vi "Test DataType Conversion.vi"() -> ()   [LabVIEW 2021]
uses:
  <vilib>/Utility/Data Type/Type Definitions/Data Type.ctl
  DataTypes_CIF_U.lvlib
  <vilib>/Utility/Data Type/NI_Data Type.lvlib
panel:
  out "Pass":bool
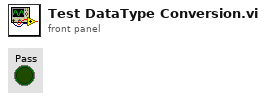
[diagram p1: front panel]
types:
  T1 = typedef "NI_Data Type.lvlib/Data Type.ctl" = enum8{"Invalid Type", "Void", "I8", "I16", "I32", "I64", "U8", "U16", "U32", "U64", "Single Float", "Double Float", "Extended Float", "Single Complex", "Double Complex", "Extended Complex", "Enum U8", "Enum U16", "Enum U32", "Enum U64", "Single Float With Unit", "Double Float With Unit", "Extended Float With Unit", "Single Complex with Unit", "Double Complex with Unit", "Extended Complex with Unit", "Boolean", "String", "Path", "Picture", "Tag", "Array", "Cluster", "Variant", "LV Variant", "Waveform", "Timestamp", "Digital Waveform", "Digital Data", "ExpressData", "Refnum", "External Data", "VI", "Poly VI", "LabVIEW Class Instance", "Fixed Point", "Set Collection", "Map Collection"}
  T2 = typedef "DataTypes_CIF_U.lvlib/Generic Datatypes.ctl" = enum16{"Invalid", "Bool", "U8", "I8", "U16", "I16", "U32", "I32", "U64", "I64", "Single Float", "Double Float", "String"}
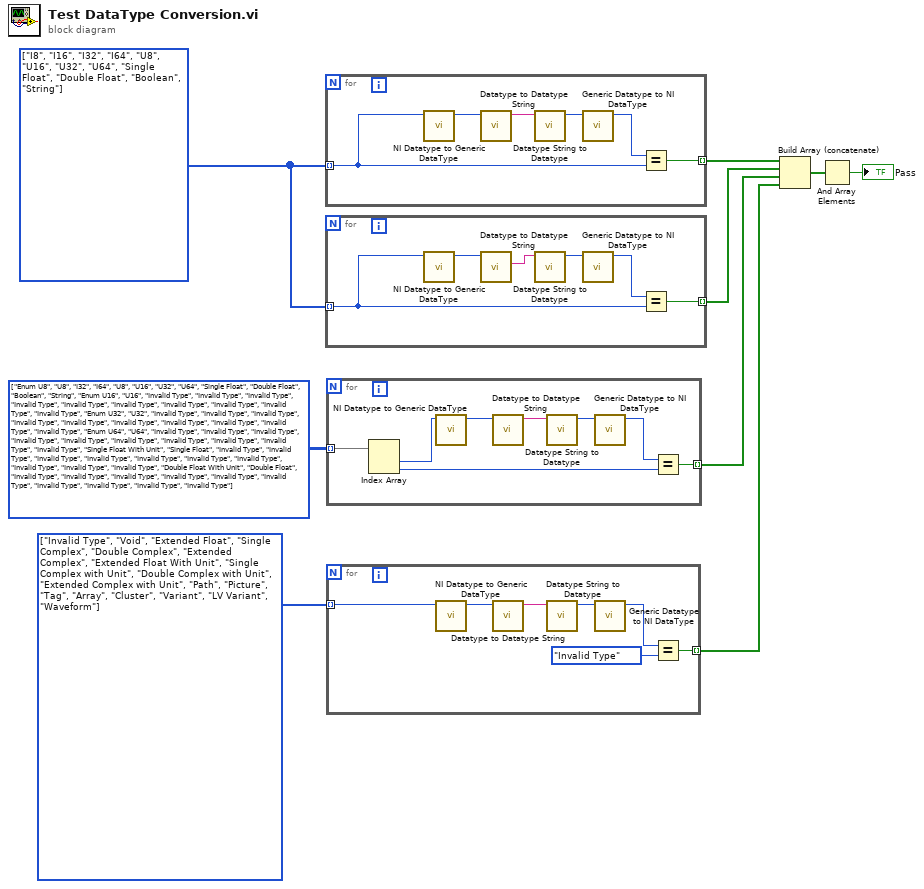
[diagram p0: block diagram]
diagram:
  w7 = T1[] [enum."Invalid Type", enum."Void", enum."Extended Float", enum."Single Complex", enum."Double Complex", enum."Extended Complex", enum."Extended Float With Unit", enum."Single Complex with Unit", enum."Double Complex with Unit", enum."Extended Complex with Unit", enum."Path", enum."Picture", enum."Tag", enum."Array", enum."Cluster", enum."Variant", enum."LV Variant", enum."Waveform"] items=["Invalid Type", "Void", "I8", "I16", "I32", "I64", "U8", "U16", "U32", "U64", "Single Float", "Double Float", "Extended Float", "Single Complex", "Double Complex", "Extended Complex", "Enum U8", "Enum U16", "Enum U32", "Enum U64", "Single Float With Unit", "Double Float With Unit", "Extended Float With Unit", "Single Complex with Unit", "Double Complex with Unit", "Extended Complex with Unit", "Boolean", "String", "Path", "Picture", "Tag", "Array", "Cluster", "Variant", "LV Variant", "Waveform", "Timestamp", "Digital Waveform", "Digital Data", "ExpressData", "Refnum", "External Data", "VI", "Poly VI", "LabVIEW Class Instance", "Fixed Point", "Set Collection", "Map Collection"]
  w8 = T1[][] [[enum."Enum U8", enum."U8", enum."I32", enum."I64", enum."U8", enum."U16", enum."U32", enum."U64", enum."Single Float", enum."Double Float", enum."Boolean", enum."String"], [enum."Enum U16", enum."U16", enum."Invalid Type", enum."Invalid Type", enum."Invalid Type", enum."Invalid Type", enum."Invalid Type", enum."Invalid Type", enum."Invalid Type", enum."Invalid Type", enum."Invalid Type", enum."Invalid Type"], [enum."Enum U32", enum."U32", enum."Invalid Type", enum."Invalid Type", enum."Invalid Type", enum."Invalid Type", enum."Invalid Type", enum."Invalid Type", enum."Invalid Type", enum."Invalid Type", enum."Invalid Type", enum."Invalid Type"], [enum."Enum U64", enum."U64", enum."Invalid Type", enum."Invalid Type", enum."Invalid Type", enum."Invalid Type", enum."Invalid Type", enum."Invalid Type", enum."Invalid Type", enum."Invalid Type", enum."Invalid Type", enum."Invalid Type"], [enum."Single Float With Unit", enum."Single Float", enum."Invalid Type", enum."Invalid Type", enum."Invalid Type", enum."Invalid Type", enum."Invalid Type", enum."Invalid Type", enum."Invalid Type", enum."Invalid Type", enum."Invalid Type", enum."Invalid Type"], [enum."Double Float With Unit", enum."Double Float", enum."Invalid Type", enum."Invalid Type", enum."Invalid Type", enum."Invalid Type", enum."Invalid Type", enum."Invalid Type", enum."Invalid Type", enum."Invalid Type", enum."Invalid Type", enum."Invalid Type"]] items=["Invalid Type", "Void", "I8", "I16", "I32", "I64", "U8", "U16", "U32", "U64", "Single Float", "Double Float", "Extended Float", "Single Complex", "Double Complex", "Extended Complex", "Enum U8", "Enum U16", "Enum U32", "Enum U64", "Single Float With Unit", "Double Float With Unit", "Extended Float With Unit", "Single Complex with Unit", "Double Complex with Unit", "Extended Complex with Unit", "Boolean", "String", "Path", "Picture", "Tag", "Array", "Cluster", "Variant", "LV Variant", "Waveform", "Timestamp", "Digital Waveform", "Digital Data", "ExpressData", "Refnum", "External Data", "VI", "Poly VI", "LabVIEW Class Instance", "Fixed Point", "Set Collection", "Map Collection"]
  w1 = T1[] [enum."I8", enum."I16", enum."I32", enum."I64", enum."U8", enum."U16", enum."U32", enum."U64", enum."Single Float", enum."Double Float", enum."Boolean", enum."String"] items=["Invalid Type", "Void", "I8", "I16", "I32", "I64", "U8", "U16", "U32", "U64", "Single Float", "Double Float", "Extended Float", "Single Complex", "Double Complex", "Extended Complex", "Enum U8", "Enum U16", "Enum U32", "Enum U64", "Single Float With Unit", "Double Float With Unit", "Extended Float With Unit", "Single Complex with Unit", "Double Complex with Unit", "Extended Complex with Unit", "Boolean", "String", "Path", "Picture", "Tag", "Array", "Cluster", "Variant", "LV Variant", "Waveform", "Timestamp", "Digital Waveform", "Digital Data", "ExpressData", "Refnum", "External Data", "VI", "Poly VI", "LabVIEW Class Instance", "Fixed Point", "Set Collection", "Map Collection"]
  n1 = for {
    tunnel: [w10] -> w6 mode=indexing
    tunnel: w1 -> [w11] mode=indexing
    n2 = call "NI Datatype to Generic DataType.vi"("NI Datatype"=w11) -> ("Generic Datatype"=w13:T2)  [unwired: 10 in]
    n3 = call "Datatype to Datatype String.vi"("Generic Datatype"=w13) -> ("String"=w14:string)  [unwired: 9 in, 1 out]
    n4 = call "Datatype String to Datatype.vi"("Datatype String"=w14) -> ("Generic Datatype"=w15:T2)  [unwired: 10 in]
    n5 = call "Generic Datatype to NI DataType.vi"("Generic Datatype"=w15) -> ("NI Datatype"=w12:T1)  [unwired: 10 in]
    n6 = Equal?(x=w12, y=w11) -> (x = y?=w10:bool)
  }
  n7 = for {
    tunnel: [w17] -> w2 mode=indexing
    tunnel: w1 -> [w18] mode=indexing
    n8 = call "NI Datatype to Generic DataType.vi"("NI Datatype"=w18) -> ("Generic Datatype"=w20:T2)  [unwired: 10 in]
    n9 = call "Datatype to Datatype String.vi"("Generic Datatype"=w20) -> ("Rust String"=w16:string)  [unwired: 9 in, 1 out]
    n10 = call "Datatype String to Datatype.vi"("Datatype String"=w16) -> ("Generic Datatype"=w21:T2)  [unwired: 10 in]
    n11 = call "Generic Datatype to NI DataType.vi"("Generic Datatype"=w21) -> ("NI Datatype"=w19:T1)  [unwired: 10 in]
    n12 = Equal?(x=w19, y=w18) -> (x = y?=w17:bool)
  }
  n13 = for {
    tunnel: [w25] -> w3 mode=indexing
    tunnel: w8 -> [w24] mode=indexing
    n14 = Index Array(array=w24) -> (element #1=w23:T1, element #2=w22:T1)  [unwired: 2 in]
    n15 = call "NI Datatype to Generic DataType.vi"("NI Datatype"=w23) -> ("Generic Datatype"=w27:T2)  [unwired: 10 in]
    n16 = call "Datatype to Datatype String.vi"("Generic Datatype"=w27) -> ("String"=w28:string)  [unwired: 9 in, 1 out]
    n17 = call "Datatype String to Datatype.vi"("Datatype String"=w28) -> ("Generic Datatype"=w29:T2)  [unwired: 10 in]
    n18 = call "Generic Datatype to NI DataType.vi"("Generic Datatype"=w29) -> ("NI Datatype"=w26:T1)  [unwired: 10 in]
    n19 = Equal?(x=w26, y=w22) -> (x = y?=w25:bool)
  }
  n20 = for {
    tunnel: [w31] -> w5 mode=indexing
    tunnel: w7 -> [w32] mode=indexing
    n21 = call "NI Datatype to Generic DataType.vi"("NI Datatype"=w32) -> ("Generic Datatype"=w34:T2)  [unwired: 10 in]
    n22 = call "Datatype to Datatype String.vi"("Generic Datatype"=w34) -> ("String"=w35:string)  [unwired: 9 in, 1 out]
    n23 = call "Datatype String to Datatype.vi"("Datatype String"=w35) -> ("Generic Datatype"=w36:T2)  [unwired: 10 in]
    n24 = call "Generic Datatype to NI DataType.vi"("Generic Datatype"=w36) -> ("NI Datatype"=w33:T1)  [unwired: 10 in]
    n25 = Equal?(x=w33, y=Data_Type."Invalid Type") -> (x = y?=w31:bool)
  }
  n26 = Build Array (concatenate)(w6, w2, w3, w5) -> (w4:bool[])
  n27 = And Array Elements(Boolean array=w4) -> (logical AND=→"Pass":bool)
